vi "Update Go To Actions.vi"(8 "Show Dialogs (default: True)":bool=TRUE, 10 "Step Update Map in":T1(c390), 11 "Settings UI in":refnum<class "Settings UI.lvclass">) -> (3 "Settings UI out":refnum<class "Settings UI.lvclass">)   [LabVIEW 2020, in "Output Sequencer.lvlib" / "Settings UI.lvclass"]
uses:
  Settings UI.lvclass
  Settings UI.lvclass/Settings UI.ctl
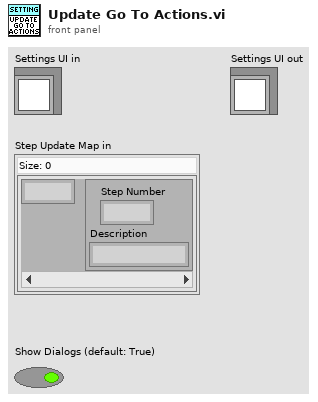
[diagram p1: front panel]
types:
  T1 = map{i32, cluster{"Step Number":i32, "Description":string}}
  T2 = typedef "Output Sequencer.lvlib/Settings UI.lvclass/Step Settings.ctl" = cluster{"Description":string, "Precondition":string, "Duration":dbl, "Mode":string, "Delay Between Values":dbl, "Analog Values":string[], "Digital Values":string[], "Postcondition":string, "On True":string, "On False":string}
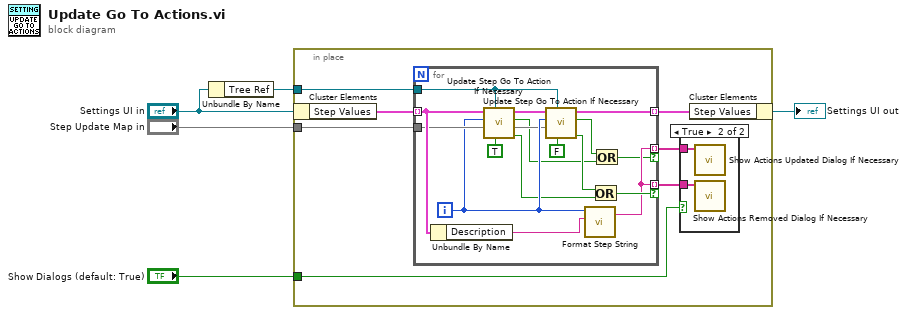
[diagram p0: block diagram]
diagram:
  n1 = Unbundle By Name("Settings UI in") -> ("Tree Ref"=w4:refnum<vi>)
  n2 = in-place {
    in-place-border: "Step Update Map in" -> [w12]
    in-place-border: w4 -> [w11]
    in-place-border: "Show Dialogs (default: True)" -> [w6]
    n3 = in-place-cluster #1("Settings UI in") -> ("Step Values"=w10:T2[])
    n4 = for {
      tunnel: w10 -> [w30] mode=indexing
      tunnel: [w20] -> w9 mode=indexing
      tunnel: w11 -> [w22]
      tunnel: w12 -> [w29]
      tunnel: [w16] -> w8 mode=indexing if=w19
      tunnel: [w16] -> w7 mode=indexing if=w15
      i -> [w26]
      n5 = Unbundle By Name(w30) -> ("Description"=w31:string)
      n6 = call "Update Step Go To Action If Necessary.vi"("Action case (T/F)"=TRUE, "TreeControl in"=w22, "Step Update Map in"=w29, "Step Number"=w26, "Step Settings in"=w30) -> ("Action removed"=w24:bool, "Step Update Map out"=w23:T1, "Action updated"=w18:bool, "Step Settings out"=w27:T2)  [unwired: 3 in]
      n7 = call "Update Step Go To Action If Necessary.vi"("Action case (T/F)"=FALSE, "TreeControl in"=w22, "Step Update Map in"=w23, "Step Number"=w26, "Step Settings in"=w27) -> ("Action removed"=w25:bool, "Action updated"=w17:bool, "Step Settings out"=w20:T2)  [unwired: 3 in, 1 out]
      n8 = call "Format Step String.vi"("Description"=w31, "Step Number"=w26) -> ("Step String out"=w16:string)  [unwired: 9 in]
      n9 = Or(x=w25, y=w24) -> (x .or. y?=w19:bool)
      n10 = Or(x=w17, y=w18) -> (x .or. y?=w15:bool)
    }
    n11 = case shown="True" w6 {
      tunnel: w8 -> [_ w14]
      tunnel: w7 -> [_ w13]
      frame False {
      }
      frame True {
        n12 = call "Show Actions Updated Dialog If Necessary.vi"("Steps with updated actions"=w13) -> ()  [unwired: 11 in]
        n13 = call "Show Actions Removed Dialog If Necessary.vi"("Steps with removed actions"=w14) -> ()  [unwired: 11 in]
      }
    }
    n14 = in-place-cluster #1("Step Values"=w9) -> (→"Settings UI out":refnum<class "Settings UI.lvclass">)
  }
